vi "GeneradorSeñales.vi"() -> ()   [LabVIEW 2020]
uses:
  <vilib>/Analysis/NI_AALPro.lvlib
panel:
  out "Waveform Graph 2":dynamicdata(graph)
  out "Waveform Graph":dbl[](graph)
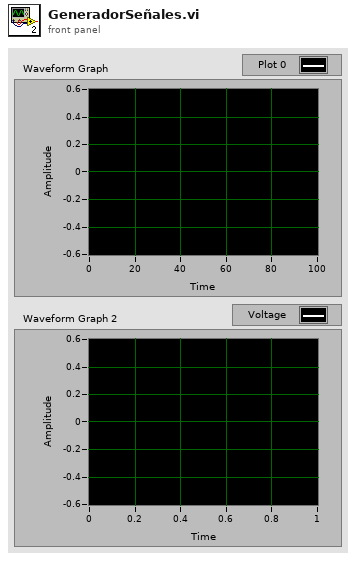
[diagram p1: front panel]
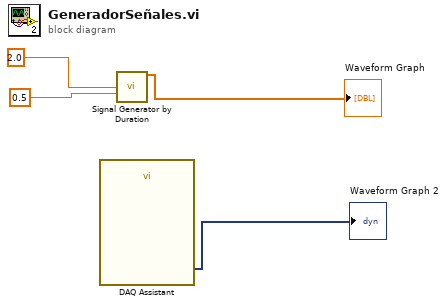
[diagram p0: block diagram]
diagram:
  n1 = call "DAQ Assistant"() -> ("data"=→"Waveform Graph 2":dynamicdata)  [unwired: 17 in, 2 out]
  n2 = call <vilib>:"Signal Generator by Duration.vi"("frequency"=2.0, "amplitude"=0.5) -> ("signal"=→"Waveform Graph":dbl[])  [unwired: 10 in, 3 out]
